vi "Helium Probe Resistance (Read).vi"(6 "ISOBUS address":T4=-1 caption="ISOBUS address (-1)", 8 "error in":errorcluster, 11 "Mercury Reference In":T5) -> (0 "error out":errorcluster, 1 "Unit":T2, 2 "Resistance Configuration":T1, 3 "Mercury Reference Out":T5, 4 "Valid?":T3)   [LabVIEW 2015, in "Mercury iXX.lvlib" / "Level Meter.lvlib"]
doc: "Returns the current resistance range of the helium probe."
uses:
  Level Meter.lvlib
  Controls/Mercury Reference.ctl
  Controls/Comms Transport Layer.ctl
  private/Controls/Query Dynamic Reference.ctl
  Controls/ISOBus Address.ctl
  Controls/Is Valid LED.ctl
  Controls/Unit String.ctl
  Controls/Resistance Configuration.ctl
  private/Controls/Command Verbs.ctl
  Mercury iXX.lvlib
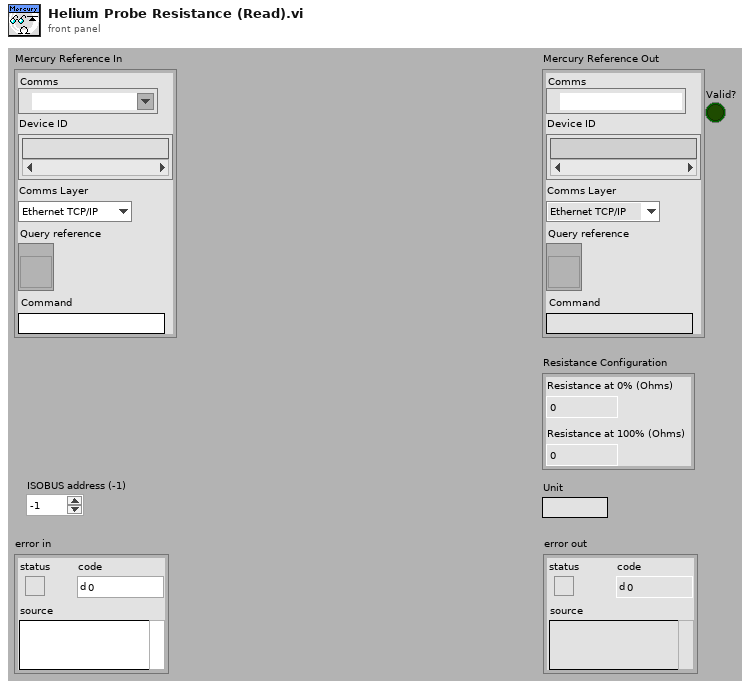
[diagram p1: front panel]
types:
  T1 = typedef "Mercury iXX.lvlib/Level Meter.lvlib/Resistance Configuration.ctl" = cluster{"Res 0%":dbl, "Res 100%":dbl}
  T2 = typedef "Mercury iXX.lvlib/Unit String.ctl" = string
  T3 = typedef "Mercury iXX.lvlib/Is Valid LED.ctl" = bool
  T4 = typedef "Mercury iXX.lvlib/ISOBus Address.ctl" = i32
  T5 = typedef "Mercury iXX.lvlib/Mercury Reference.ctl" = cluster{"Comms":refnum<visa-resource-name>, "Device ID":string[], "Comms Layer":T6, "Command":string, "Query reference":T7}
  T6 = typedef "Mercury iXX.lvlib/Comms Transport Layer.ctl" = enum16{"Ethernet TCP/IP", "USB", "ISOBus - RS-232", "GPIB"}
  T7 = typedef "Mercury iXX.lvlib/Query Dynamic Reference.ctl" = refnum<vi>
  T8 = typedef "Mercury iXX.lvlib/Command Verbs.ctl" = string
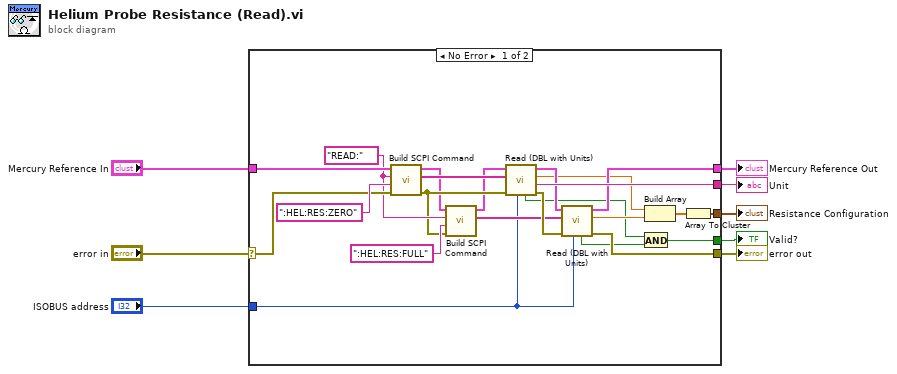
[diagram p0: block diagram]
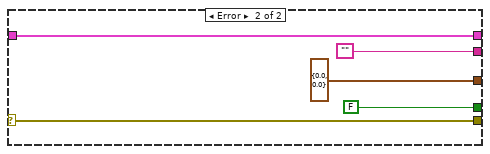
[diagram p2: hidden frame]
diagram:
  n1 = case shown="No Error" "error in" {
    selector: "error in" -> [w27 w35]
    tunnel: "Mercury Reference In" -> [w28 w36]
    tunnel: [w18 w36] -> w5
    tunnel: [w20 w35] -> w1
    tunnel: "ISOBUS address" -> [w9 _]
    tunnel: [w29 ""] -> w3
    tunnel: [w10 FALSE ("Valid?")] -> w2
    tunnel: [w11 cluster{"[0]":dbl, "[1]":dbl} {"[0]"=0.0, "[1]"=0.0}] -> w4
    frame No Error {
      w25 = T8 "READ:" ("Verb")
      n2 = call "Build SCPI Command.vi"("error in"=w27, "Noun(s)"=":HEL:RES:ZERO" ("Command"), "Verb"=w25, "Mercury Reference In"=w28) -> ("error out"=w24:errorcluster, "SCPI Message(s)"=w30:string[], "Mercury Reference Out"=w23:T5)  [unwired: 5 out]
      n3 = call "Build SCPI Command.vi"("error in"=w24, "Noun(s)"=":HEL:RES:FULL" ("Command"), "Verb"=w25, "Mercury Reference In"=w23) -> ("SCPI Message(s)"=w17:string[], "Mercury Reference Out"=w22:T5)  [unwired: 6 out]
      n4 = call "Read (DBL with Units).vi"("ISOBUS address"=w9, "error in"=w24, "SCPI Message(s)"=w30, "Mercury Reference In"=w22) -> ("error out"=w21:errorcluster, "Unit"=w29:T2, "Data (Dbl)"=w16:dbl, "Mercury Reference Out"=w19:T5, "Valid?"=w14:T3)  [unwired: 3 out]
      n5 = call "Read (DBL with Units).vi"("ISOBUS address"=w9, "error in"=w21, "SCPI Message(s)"=w17, "Mercury Reference In"=w19) -> ("error out"=w20:errorcluster, "Data (Dbl)"=w15:dbl, "Mercury Reference Out"=w18:T5, "Valid?"=w13:T3)  [unwired: 4 out]
      n6 = And(x=w14, y=w13) -> (x .and. y?=w10:T3)
      n7 = Build Array(w16, w15) -> (w12:dbl[])
      n8 = Array To Cluster(array=w12) -> (cluster=w11:cluster{"[0]":dbl, "[1]":dbl})
    }
    frame Error {
    }
  }
  "Mercury Reference Out" <- w5
  "error out" <- w1
  "Valid?" <- w2
  "Unit" <- w3
  "Resistance Configuration" <- w4
